vi "Destoy queue.vi"(8 "error in":errorcluster, 11 "queue in":refnum<queue>) -> (0 "error out":errorcluster)   [LabVIEW 2025, in "Queue API.lvlib"]
uses:
  Queue API.lvlib
  Controls/CAN Sending Data.ctl
  Controls/CAN Payload.ctl
  Commands.ctl
  Notifier Data.ctl
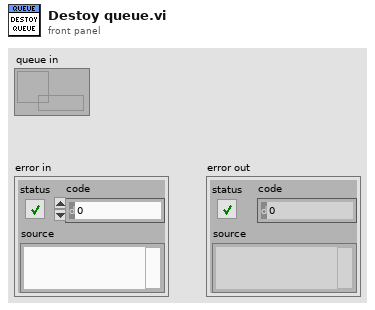
[diagram p1: front panel]
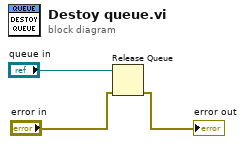
[diagram p0: block diagram]
diagram:
  n1 = Release Queue(queue="queue in", error in (no error)="error in") -> (error out=→"error out":errorcluster)  [unwired: 1 in, 2 out]
